vi "Periodic Tasks.vi"(8 "error in":errorcluster) -> ()   [LabVIEW 2017]
doc: "This VI runs in parallel to other tasks. It can contain as many user-defined periodic loops as you need. These can carry out PID or other sorts of timed response."
uses:
  <vilib>/Rock Robotics/WPI/DriverStation/WPI_DriverStationAllianceInfo.ctl
  <vilib>/Rock Robotics/WPI/ThirdParty/Sensors/navX/_TypeDefs/FRIC_navX_DeviceNumbersTypeDef.ctl
  Lift States.ctl
  Robot Global Data.vi
  <vilib>/Rock Robotics/WPI/Utilities/WPI_GetSetVariantRefNum.vi
panel:
  in  "Red Alliance":bool
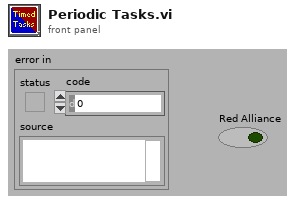
[diagram p1: front panel]
types:
  T1 = typedef "WPI_MotorControlDeviceRef.ctl" = cluster{"DeviceStatus":errorcluster, "Type":T2, "PWM":cluster{"PWM Channel":T3, "DeadBand":T4}, "CAN":cluster{"Device Number":u8, "SetOutput VI Ref":variant, "GetOutput VI Ref":variant, "Enable VI Ref":variant, "Disable VI Ref":variant, "Data":variant}, "Invert":bool, "DIO PWM":cluster{"PWM \"Enable\" Channel":T3, "DIOChannel":T5, "PWM Rate":dbl}}
  T2 = typedef "WPI_MotorControlType.ctl" = enum16{"PWM", "CAN", "DIO PWM"}
  T3 = typedef "FPGA_DIOPWMChannel.ctl" = enum8{"PWM 0", "PWM 1", "PWM 2", "PWM 3", "PWM 4", "PWM 5", "PWM 6", "PWM 7", "PWM 8", "PWM 9", "PWM MXP 0", "PWM MXP 1", "PWM MXP 2", "PWM MXP 3", "PWM MXP 4", "PWM MXP 5", "PWM MXP 6", "PWM MXP 7", "PWM MXP 8", "PWM MXP 9", "Invalid"}
  T4 = typedef "WPI_PWMDeadband.ctl" = cluster{"Name":string, "maxPositivePwm":i32, "minPositivePwm":i32, "centerPwm":i32, "maxNegativePwm":i32, "minNegativePwm":i32, "angularRange":u16}
  T5 = typedef "FPGA_DIOChannel.ctl" = enum8{"DIO 0", "DIO 1", "DIO 2", "DIO 3", "DIO 4", "DIO 5", "DIO 6", "DIO 7", "DIO 8", "DIO 9", "DIO MXP 0", "DIO MXP 1", "DIO MXP 2", "DIO MXP 3", "DIO MXP 4", "DIO MXP 5", "DIO MXP 6", "DIO MXP 7", "DIO MXP 8", "DIO MXP 9", "DIO MXP 10", "DIO MXP 11", "DIO MXP 12", "DIO MXP 13", "DIO MXP 14", "DIO MXP 15", "SPI Port CS1", "SPI Port CS2", "SPI Port CS3", "SPI Port MISO", "SPI Port MOSI", "Invalid"}
  T6 = typedef "WPI_SolenoidDevRef.ctl" = cluster{"DevStatus":errorcluster, "Pneumatics Control Module":u8, "Forward Solenoid Channel":T7, "Reverse Solenoid Channel":T7}
  T7 = typedef "WPI_SolenoidChannel.ctl" = enum8{"Solenoid 0", "Solenoid 1", "Solenoid 2", "Solenoid 3", "Solenoid 4", "Solenoid 5", "Solenoid 6", "Solenoid 7", "Invalid"}
  T8 = typedef "WPI_JoystickDevRef.ctl" = cluster{"Device":T9}
  T9 = typedef "WPI_JoystickDeviceEnum.ctl" = enum16{"USB 0", "USB 1", "USB 2", "USB 3", "USB 4", "USB 5"}
  T10 = typedef "WPI_DigitalInputDevRef.ctl" = cluster{"DevStatus":errorcluster, "DIO Channel":T5}
  T11 = typedef "WPI_AnalogChannelDevRef.ctl" = cluster{"DevStatus":errorcluster, "Analog Channel":T12}
  T12 = typedef "FPGA_AIChannel.ctl" = enum8{"AI 0", "AI 1", "AI 2", "AI 3", "AI MXP 0", "AI MXP 1", "AI MXP 2", "AI MXP 3", "Invalid"}
  T13 = typedef "WPI_EncoderDevRef.ctl" = cluster{"DevStatus":errorcluster, "EncoderIndex":T14, "CounterIndex":T15, "DistancePerCount":dbl, "Decoding Type":T16}
  T14 = typedef "FPGA_EncoderIdx.ctl" = enum8{"Enc 0", "Enc 1", "Enc 2", "Enc 3", "Enc 4", "Enc 5", "Enc 6", "Enc 7", "Invalid"}
  T15 = typedef "FPGA_CounterCtrSystemIndex.ctl" = enum8{"Ctr 0", "Ctr 1", "Ctr 2", "Ctr 3", "Ctr 4", "Ctr 5", "Ctr 6", "Ctr 7", "Invalid"}
  T16 = typedef "WPI_EncoderType.ctl" = enum16{"1x", "2x", "4x"}
  T17 = cluster{"MotorControlDevRef":T1, "MotorControlDevRef":T1, "SolenoidDevRef":T6, "MotorControlDevRef":T1, "MotorControlDevRef":T1, "MotorControlDevRef":T1, "SolenoidDevRef":T6, "SolenoidDevRef":T6, "SolenoidDevRef":T6, "MotorControlDevRef":T1}
  T18 = typedef "WPI_I2CDevRef.ctl" = cluster{"DevStatus":errorcluster, "Device Address":u8, "Handle":i32, "I2C Bus":T19}
  T19 = typedef "i2c_bus.ctl" = enum16{"I2C On-Board", "I2C MXP", "Invalid"}
  T20 = cluster{"JoystickDevRef":T8, "JoystickDevRef":T8, "JoystickDevRef":T8, "JoystickDevRef":T8}
  T21 = typedef "FRIC_navX_DeviceNumbersTypeDef.ctl" = enum16{"Dev0", "Dev1", "Dev2", "Dev3"}
  T22 = cluster{"Yaw":dbl, "Roll":dbl, "Pitch":dbl, "Heading":dbl, "Fused Heading":dbl}
  T23 = typedef "WPI_DriverStationAllianceInfo.ctl" = enum16{"Red", "Blue", "Invalid"}
  T24 = typedef "Lift States.ctl" = enum16{"Manual", "Scale Low", "Scale Middle", "Scale High", "Rock Bottom", "Almost Down"}
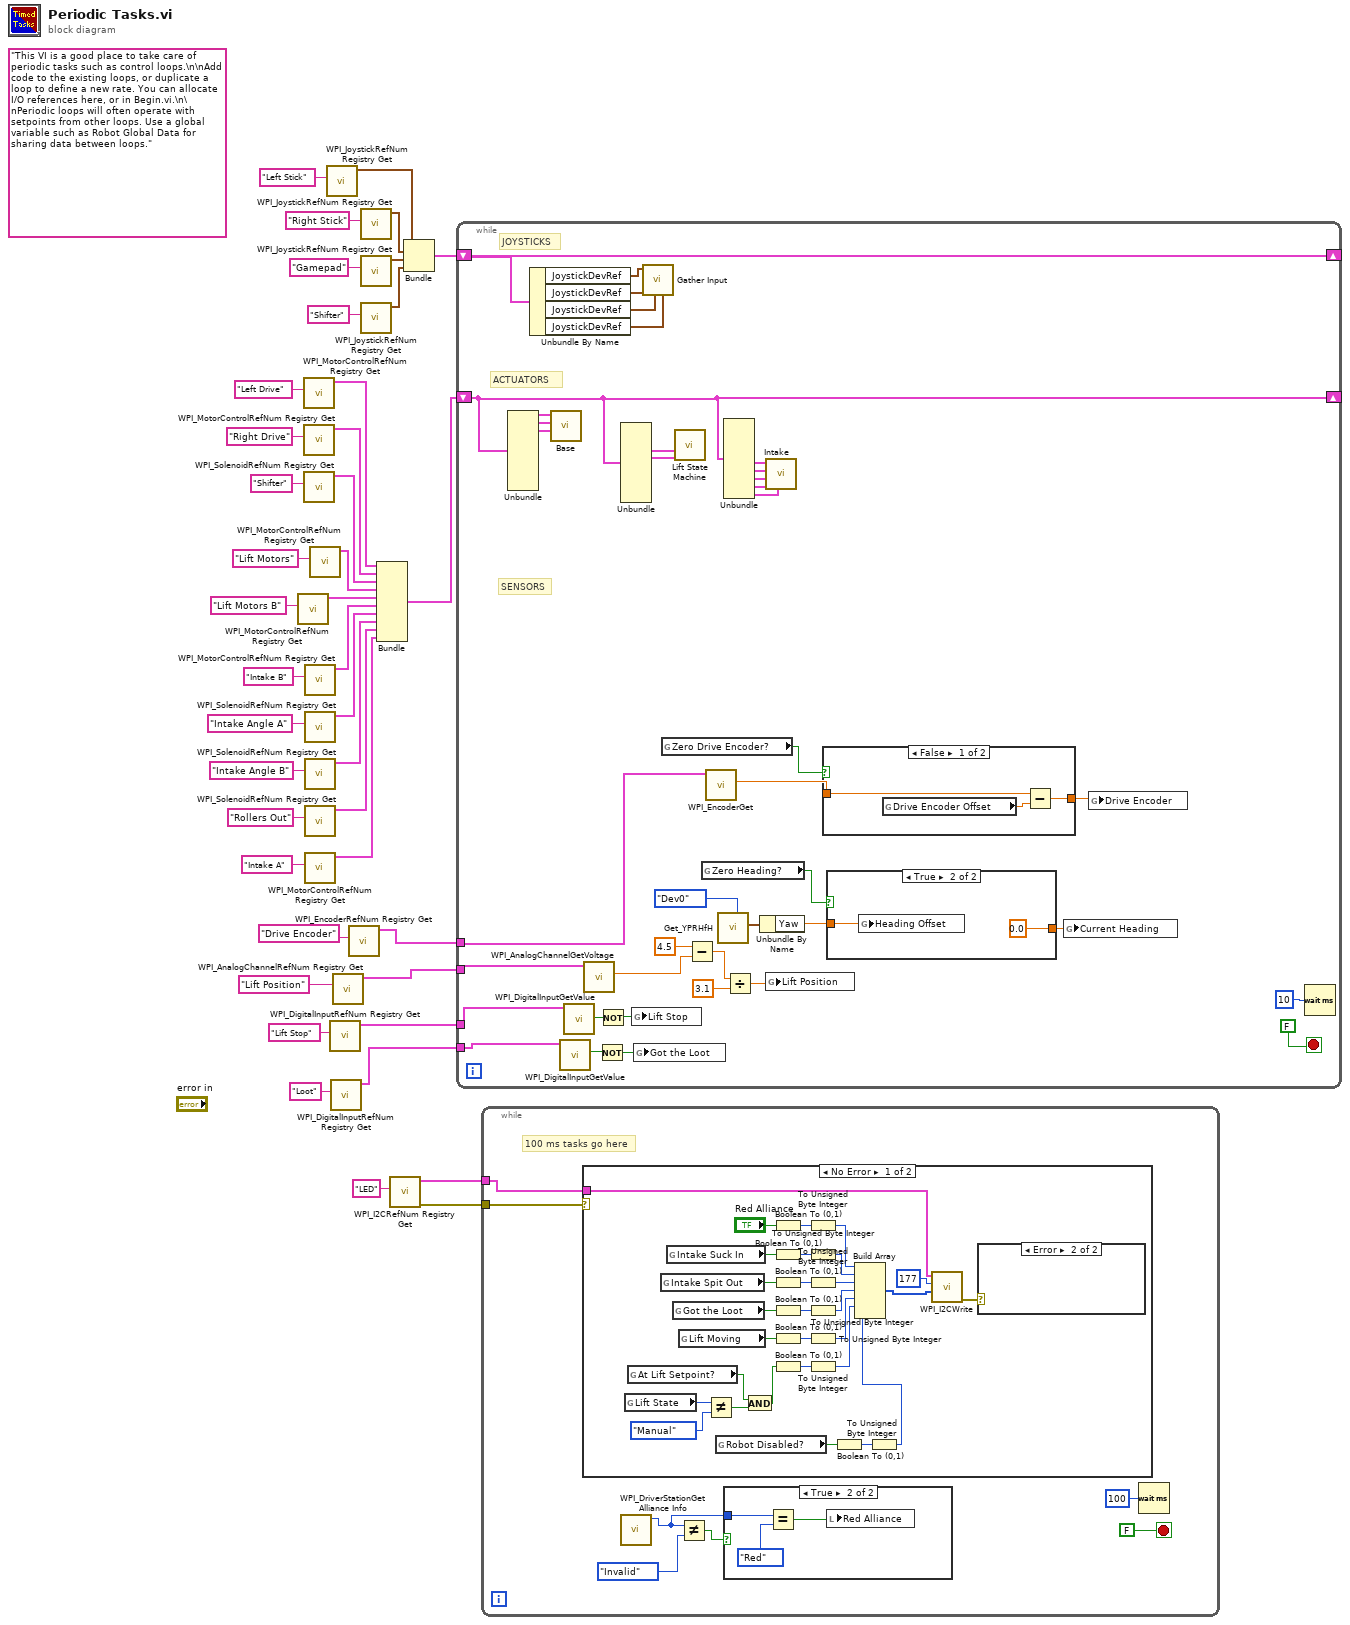
[diagram p0: block diagram]
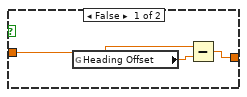
[diagram p5: hidden frame]
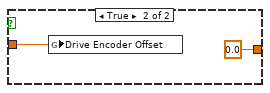
[diagram p6: hidden frame]
diagram:
  (unwired) "This VI is a good place to take care of periodic tasks such as control loops.\n\nAdd code to the existing loops, or duplicate a loop to define a new rate. You can allocate I/O references here, or in Begin.vi.\n\nPeriodic loops will often operate with setpoints from other loops. Use a global variable such as Robot Global Data for sharing data between loops."
  n1 = call <vilib>:"WPI_MotorControlRefNum Registry Get.vi"("refnum name"="Lift Motors B") -> ("MotorControlDevRef"=w16:T1)  [unwired: 9 in, 1 out]
  n2 = call <vilib>:"WPI_MotorControlRefNum Registry Get.vi"("refnum name"="Left Drive") -> ("MotorControlDevRef"=w38:T1)  [unwired: 9 in, 1 out]
  n3 = call <vilib>:"WPI_MotorControlRefNum Registry Get.vi"("refnum name"="Right Drive") -> ("MotorControlDevRef"=w37:T1)  [unwired: 9 in, 1 out]
  n4 = call <vilib>:"WPI_SolenoidRefNum Registry Get.vi"("refnum name"="Shifter") -> ("SolenoidDevRef"=w27:T6)  [unwired: 9 in, 1 out]
  n5 = call <vilib>:"WPI_MotorControlRefNum Registry Get.vi"("refnum name"="Intake B") -> ("MotorControlDevRef"=w31:T1)  [unwired: 9 in, 1 out]
  n6 = call <vilib>:"WPI_SolenoidRefNum Registry Get.vi"("refnum name"="Intake Angle A") -> ("SolenoidDevRef"=w30:T6)  [unwired: 9 in, 1 out]
  n7 = call <vilib>:"WPI_SolenoidRefNum Registry Get.vi"("refnum name"="Intake Angle B") -> ("SolenoidDevRef"=w29:T6)  [unwired: 9 in, 1 out]
  n8 = call <vilib>:"WPI_SolenoidRefNum Registry Get.vi"("refnum name"="Rollers Out") -> ("SolenoidDevRef"=w20:T6)  [unwired: 9 in, 1 out]
  n9 = call <vilib>:"WPI_MotorControlRefNum Registry Get.vi"("refnum name"="Intake A") -> ("MotorControlDevRef"=w18:T1)  [unwired: 9 in, 1 out]
  n10 = call <vilib>:"WPI_MotorControlRefNum Registry Get.vi"("refnum name"="Lift Motors") -> ("MotorControlDevRef"=w26:T1)  [unwired: 9 in, 1 out]
  n11 = call <vilib>:"WPI_JoystickRefNum Registry Get.vi"("refnum name"="Left Stick") -> ("JoystickDevRef"=w6:T8)  [unwired: 9 in, 1 out]
  n12 = call <vilib>:"WPI_DigitalInputRefNum Registry Get.vi"("refnum name"="Lift Stop") -> ("DigitalInputDevRef"=w11:T10)  [unwired: 9 in, 1 out]
  n13 = call <vilib>:"WPI_DigitalInputRefNum Registry Get.vi"("refnum name"="Loot") -> ("DigitalInputDevRef"=w1:T10)  [unwired: 9 in, 1 out]
  n14 = call <vilib>:"WPI_AnalogChannelRefNum Registry Get.vi"("refnum name"="Lift Position") -> ("AIDeviceRef"=w22:T11)  [unwired: 9 in, 1 out]
  n15 = call <vilib>:"WPI_EncoderRefNum Registry Get.vi"("refnum name"="Drive Encoder") -> ("EncoderDevRef"=w23:T13)  [unwired: 9 in, 1 out]
  n16 = call <vilib>:"WPI_JoystickRefNum Registry Get.vi"("refnum name"="Right Stick") -> ("JoystickDevRef"=w5:T8)  [unwired: 9 in, 1 out]
  n17 = call <vilib>:"WPI_JoystickRefNum Registry Get.vi"("refnum name"="Gamepad") -> ("JoystickDevRef"=w4:T8)  [unwired: 9 in, 1 out]
  n18 = call <vilib>:"WPI_JoystickRefNum Registry Get.vi"("refnum name"="Shifter") -> ("JoystickDevRef"=w3:T8)  [unwired: 9 in, 1 out]
  n19 = Bundle("MotorControlDevRef"=w38, "MotorControlDevRef"=w37, "SolenoidDevRef"=w27, "MotorControlDevRef"=w26, "MotorControlDevRef"=w16, "MotorControlDevRef"=w31, "SolenoidDevRef"=w30, "SolenoidDevRef"=w29, "SolenoidDevRef"=w20, "MotorControlDevRef"=w18) -> (w36:T17)  [unwired: 1 in]
  n20 = call <vilib>:"WPI_I2CRefNum Registry Get.vi"("refnum name"="LED") -> ("error out"=w13:errorcluster, "I2CDevRef"=w14:T18)  [unwired: 9 in]
  n21 = Bundle("JoystickDevRef"=w6, "JoystickDevRef"=w5, "JoystickDevRef"=w4, "JoystickDevRef"=w3) -> (w41:T20)  [unwired: 1 out]
  n22 = while {
    shift-right: [w78] -> _
    shift-left: w41 -> [w78]
    shift-right: [w65] -> _
    shift-left: w36 -> [w65]
    tunnel: w23 -> [w57]
    tunnel: w22 -> [w56]
    tunnel: w11 -> [w52]
    tunnel: w1 -> [w46]
    stop <- FALSE stop-if-true
    # "SENSORS"
    # "JOYSTICKS"
    # "ACTUATORS"
    n23 = Unbundle(w65) -> ("MotorControlDevRef"=w64:T1, "MotorControlDevRef"=w63:T1, "SolenoidDevRef"=w62:T6)  [unwired: 7 out]
    n24 = Unbundle By Name(w78) -> ("JoystickDevRef"=w77:T8, "JoystickDevRef"=w76:T8, "JoystickDevRef"=w74:T8, "JoystickDevRef"=w75:T8)
    n25 = call "Base.vi"("Shifter"=w62, "Right Drive"=w63, "Left Drive"=w64) -> ()  [unwired: 9 in]
    n26 = call <vilib>:"WPI_DigitalInputGetValue.vi"("DigitalInputDevRef"=w46) -> ("Value"=w43:bool)  [unwired: 8 in, 2 out]
    n27 = call <vilib>:"WPI_DigitalInputGetValue.vi"("DigitalInputDevRef"=w52) -> ("Value"=w45:bool)  [unwired: 8 in, 2 out]
    n28 = call <vilib>:"WPI_AnalogChannelGetVoltage.vi"("AIDeviceRef"=w56) -> ("Voltage"=w50:dbl)  [unwired: 8 in, 2 out]
    n29 = Not(x=w43) -> (.not. x?=w42:bool)
    n30 = Not(x=w45) -> (.not. x?=w44:bool)
    n31 = Unbundle(w65) -> ("MotorControlDevRef"=w58:T1, "MotorControlDevRef"=w53:T1)  [unwired: 8 out]
    n32 = global write "Robot Global Data.vi" "Lift Stop"(w44) -> ()
    n33 = global write "Robot Global Data.vi" "Got the Loot"(w42) -> ()
    n34 = call "Gather Input.vi"("Shifter"=w75, "Gamepad"=w74, "Joystick Right"=w76, "Joystick Left"=w77) -> ()  [unwired: 8 in]
    n35 = global read "Robot Global Data.vi" "Zero Drive Encoder?"() -> (w73:bool)
    n36 = call "Lift State Machine.vi"("Lift Motors B"=w53, "Lift Motors"=w58) -> ()  [unwired: 10 in]
    n37 = Subtract(x=4.5, y=w50) -> (x-y=w49:dbl)
    n38 = global read "Robot Global Data.vi" "Zero Heading?"() -> (w70:bool)
    n39 = call <vilib>:"WPI_EncoderGet.vi"("EncoderDevRef"=w57) -> ("Distance"=w72:dbl)  [unwired: 5 in, 5 out]
    n40 = call <vilib>:"Get_YPRHfH.vi"("Device Number"=FRIC_navX_DeviceNumbersTypeDef."Dev0") -> ("YRPHfH"=w69:T22)  [unwired: 10 in]
    n41 = Unbundle(w65) -> ("MotorControlDevRef"=w61:T1, "SolenoidDevRef"=w60:T6, "SolenoidDevRef"=w59:T6, "SolenoidDevRef"=w55:T6, "MotorControlDevRef"=w54:T1)  [unwired: 5 out]
    n42 = Divide(x=w49, y=3.1) -> (x/y=w47:dbl)
    n43 = Unbundle By Name(w69) -> ("Yaw"=w68:dbl)
    n44 = call "Intake.vi"("Motor A"=w54, "Rollers Out"=w55, "Intake Angle B"=w59, "Intake Angle A"=w60, "Motor B"=w61) -> ()  [unwired: 7 in]
    n45 = global write "Robot Global Data.vi" "Lift Position"(w47) -> ()
    n46 = case shown="False" w73 {
      tunnel: [w87 0.0] -> w71
      tunnel: w72 -> [w86 w90]
      frame False {
        n47 = global read "Robot Global Data.vi" "Drive Encoder Offset"() -> (w88:dbl)
        n48 = Subtract(x=w86, y=w88) -> (x-y=w87:dbl)
      }
      frame True {
        n49 = global write "Robot Global Data.vi" "Drive Encoder Offset"(w90) -> ()
      }
    }
    n50 = case shown="True" w70 {
      tunnel: w68 -> [w83 w85]
      tunnel: [w81 0.0] -> w67
      frame False {
        n51 = global read "Robot Global Data.vi" "Heading Offset"() -> (w82:dbl)
        n52 = Subtract(x=w83, y=w82) -> (x-y=w81:dbl)
      }
      frame True {
        n53 = global write "Robot Global Data.vi" "Heading Offset"(w85) -> ()
      }
    }
    n54 = global write "Robot Global Data.vi" "Current Heading"(w67) -> ()
    n55 = global write "Robot Global Data.vi" "Drive Encoder"(w71) -> ()
    n56 = Wait (ms)(milliseconds to wait=u32 10) -> ()  [unwired: 1 out]
  }
  n57 = while {
    tunnel: w14 -> [w94]
    tunnel: w13 -> [w95]
    stop <- FALSE stop-if-true
    # "100 ms tasks go here"
    n58 = case shown="No Error" w95 {
      tunnel: w94 -> [w125 _]
      frame No Error {
        n59 = global read "Robot Global Data.vi" "Lift State"() -> (w108:T24)
        n60 = global read "Robot Global Data.vi" "At Lift Setpoint?"() -> (w105:bool)
        n61 = global read "Robot Global Data.vi" "Intake Spit Out"() -> (w115:bool)
        n62 = global read "Robot Global Data.vi" "Intake Suck In"() -> (w114:bool)
        n63 = global read "Robot Global Data.vi" "Got the Loot"() -> (w116:bool)
        n64 = global read "Robot Global Data.vi" "Lift Moving"() -> (w111:bool)
        n65 = Not Equal?(x=w108, y=Lift_States."Manual") -> (x != y?=w104:bool)
        n66 = global read "Robot Global Data.vi" "Robot Disabled?"() -> (w103:bool)
        n67 = And(x=w105, y=w104) -> (x .and. y?=w106:bool)
        n68 = Boolean To (0,1)(Boolean="Red Alliance") -> (0, 1=w122:i16)
        n69 = Boolean To (0,1)(Boolean=w114) -> (0, 1=w121:i16)
        n70 = Boolean To (0,1)(Boolean=w115) -> (0, 1=w120:i16)
        n71 = Boolean To (0,1)(Boolean=w116) -> (0, 1=w119:i16)
        n72 = Boolean To (0,1)(Boolean=w111) -> (0, 1=w113:i16)
        n73 = Boolean To (0,1)(Boolean=w106) -> (0, 1=w110:i16)
        n74 = To Unsigned Byte Integer(number=w122) -> (unsigned 8bit integer=w129:u8)
        n75 = To Unsigned Byte Integer(number=w121) -> (unsigned 8bit integer=w128:u8)
        n76 = To Unsigned Byte Integer(number=w120) -> (unsigned 8bit integer=w118:u8)
        n77 = To Unsigned Byte Integer(number=w119) -> (unsigned 8bit integer=w117:u8)
        n78 = To Unsigned Byte Integer(number=w113) -> (unsigned 8bit integer=w112:u8)
        n79 = To Unsigned Byte Integer(number=w110) -> (unsigned 8bit integer=w109:u8)
        n80 = Boolean To (0,1)(Boolean=w103) -> (0, 1=w102:i16)
        n81 = To Unsigned Byte Integer(number=w102) -> (unsigned 8bit integer=w101:u8)
        n82 = Build Array(w129, w128, w118, w117, w112, w109, w101) -> (w127:u8[])
        n83 = call <vilib>:"WPI_I2CWrite.vi"("I2CDataToSend"=w127, "I2CRegister"=u8 177, "I2CDevRef"=w125) -> ("error out"=w124:errorcluster)  [unwired: 7 in, 1 out]
        n84 = case shown="Error" w124 {
          frame No Error {
          }
          frame Error {
          }
        }
      }
      frame Error {
      }
    }
    n85 = call <vilib>:"WPI_DriverStationGet Alliance Info.vi"() -> ("Alliance"=w91:T23)  [unwired: 6 in, 5 out]
    n86 = Not Equal?(x=w91, y=WPI_DriverStationAllianceInfo."Invalid") -> (x != y?=w92:bool)
    n87 = case shown="True" w92 {
      tunnel: w91 -> [_ w100]
      frame False {
      }
      frame True {
        n88 = Equal?(x=w100, y=WPI_DriverStationAllianceInfo."Red" ("x")) -> (x = y?=w98:bool)
        n89 = local write "Red Alliance"(w98) -> ()
      }
    }
    n90 = Wait (ms)(milliseconds to wait=u32 100) -> ()  [unwired: 1 out]
  }
